vi "RoomParamsStack.vi"(8 "error in (no error)":errorcluster, 11 "RoomNumber":i32) -> (0 "error out":errorcluster, 2 "HierarchyParams":variant[](array[variant]), 3 "Room":refnum<class "Room.lvclass">)   [LabVIEW 2020, in "Room.lvclass"]
uses:
  Room.lvclass
  Protected/property/Read RoomParams.vi
  Room.lvclass/Room.ctl
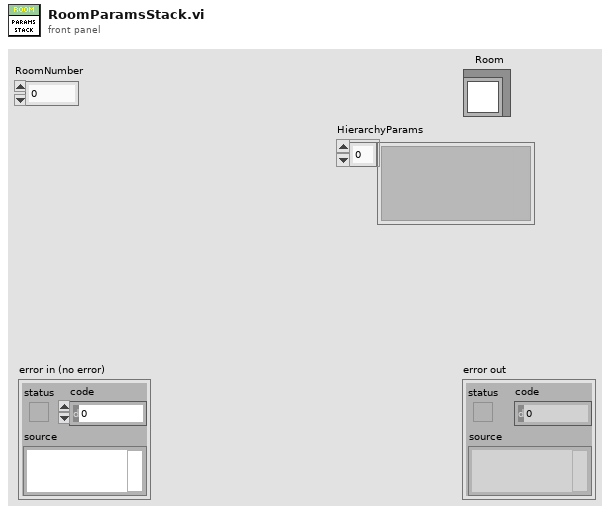
[diagram p1: front panel]
types:
  T1 = typedef "Room.lvclass/RoomParams.ctl" = cluster{"roomNumber":i32}
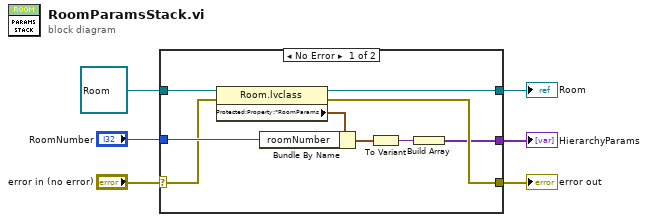
[diagram p0: block diagram]
diagram:
  n1 = case shown="No Error" "error in (no error)" {
    selector: "error in (no error)" -> [w7 w17]
    tunnel: [w13 w17] -> w5
    tunnel: refnum<class "Room.lvclass"> refnum ("Milk") -> [w15 w16]
    tunnel: [w14 w16] -> w3
    tunnel: [w12 _] -> w2
    tunnel: "RoomNumber" -> [w11 _]
    frame No Error {
      n2 = property class="Room.lvclass"(reference=w15, error in=w7) -> (reference out=w14:refnum<class "Room.lvclass">, error out=w13:errorcluster, "Protected:Property:*RoomParams"=w8:T1)
      n3 = Bundle By Name(cluster=w8, "roomNumber"=w11) -> (w10:T1)
      n4 = To Variant(anything=w10) -> (Variant=w9:variant)
      n5 = Build Array(w9) -> (w12:variant[])
    }
    frame Error {
    }
  }
  "error out" <- w5
  "Room" <- w3
  "HierarchyParams" <- w2
